vi "ConvStringIntoArrayString(SubVI).vi"(8 "Error In":errorcluster, 11 "String In":string) -> (0 "Error Out":errorcluster, 3 "Array String Out":string[](array[string]))   [LabVIEW 2018]
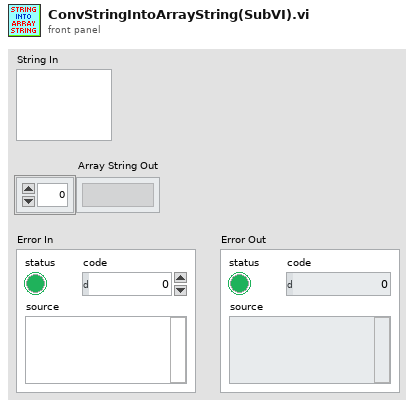
[diagram p1: front panel]
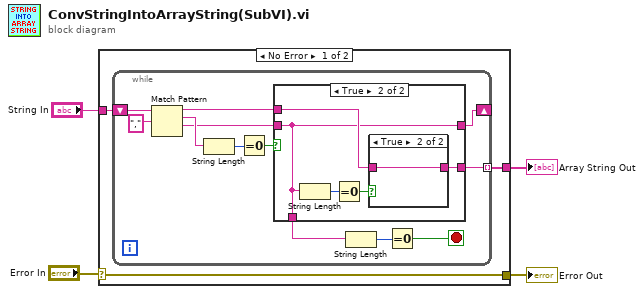
[diagram p0: block diagram]
diagram:
  n1 = case shown="No Error" "Error In" {
    selector: "Error In" -> [w5 w28]
    tunnel: "String In" -> [w7 _]
    tunnel: [w6 _] -> w3
    tunnel: [w5 w28] -> w1
    frame No Error {
      n2 = while {
        shift-right: [w15] -> _
        shift-left: w7 -> [w19]
        tunnel: [w8] -> w6 mode=indexing
        stop <- w10 stop-if-true
        n3 = Match Pattern(string=w19, regular expression="," ("string")) -> (before substring=w13:string, match substring=w17:string, after substring=w14:string)  [unwired: 1 in, 1 out]
        n4 = String Length(string=w17) -> (length=w18:i32)
        n5 = Equal To 0?(x=w18) -> (x = 0?=w16:bool)
        n6 = case shown="True" w16 {
          tunnel: [w21 w23] -> w15
          tunnel: w14 -> [w21 w23]
          tunnel: w13 -> [w20 w24]
          tunnel: [w21 w23] -> w12
          tunnel: [w20 w22] -> w8
          frame False {
          }
          frame True {
            n7 = String Length(string=w23) -> (length=w25:i32)
            n8 = Equal To 0?(x=w25) -> (x = 0?=w26:bool)
            n9 = case shown="True" w26 {
              tunnel: [_ w27] -> w22
              tunnel: w24 -> [_ w27]
              frame False {
              }
              frame True {
              }
            }
          }
        }
        n10 = String Length(string=w12) -> (length=w11:i32)
        n11 = Equal To 0?(x=w11) -> (x = 0?=w10:bool)
      }
    }
    frame Error {
    }
  }
  "Array String Out" <- w3
  "Error Out" <- w1
